vi "Read frames.vi"(9 "FlatSequence in":refnum<class "FlatSequence.lvclass">) -> (3 "FlatSequence out":refnum<class "FlatSequence.lvclass">, 4 "frames":refnum<class "FlatSequenceFrame.lvclass">[](array[class]))   [LabVIEW 2014, in "FlatSequence.lvclass"]
uses:
  FlatSequence.lvclass
  FlatSequenceFrame/FlatSequenceFrame.lvclass
  FlatSequence.lvclass/FlatSequence.ctl
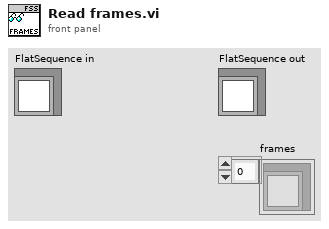
[diagram p1: front panel]
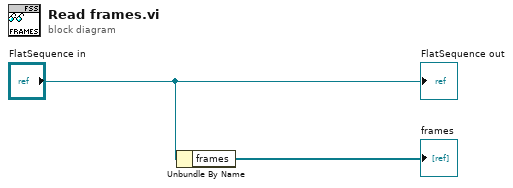
[diagram p0: block diagram]
diagram:
  n1 = Unbundle By Name("FlatSequence in") -> ("frames"=→"frames":refnum<class "FlatSequenceFrame.lvclass">[])
  "FlatSequence out" <- "FlatSequence in"
